vi "ArmEndEffectorPosition.vi"(2 "Wrist Angle (deg)":dbl, 3 "Elbow Angle (deg)":dbl, 4 "Shoulder Angle (deg)":dbl) -> (0 "Rotation Vector (deg)":cluster{"roll":dbl, "pitch":dbl, "yaw":dbl}, 1 "Translation Vector (in)":dbl[](array[numeric]))   [LabVIEW 2020]
doc: "Calculates the goal end effector position based on the goal arm joint angles."
uses:
  GlobalArm.vi
  <vilib>/robotics/Kinematics/Robot/Forward Kinematics (Point).vi
  <vilib>/robotics/Kinematics/NI_Kinematics.lvlib
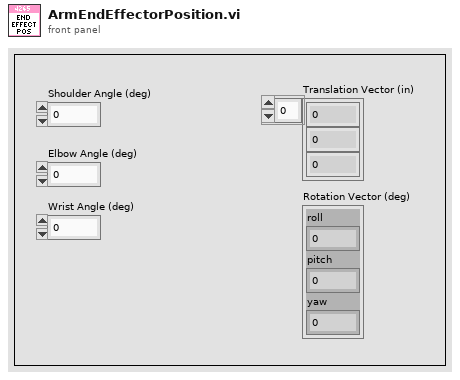
[diagram p1: front panel]
types:
  T1 = typedef "NI_Matrix.lvlib/RealMatrix.ctl" = dbl[][]
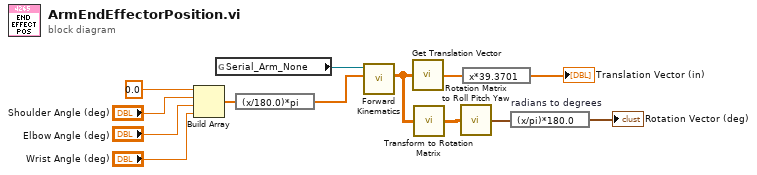
[diagram p0: block diagram]
diagram:
  n1 = Build Array(0.0 ("element"), "Shoulder Angle (deg)", "Elbow Angle (deg)", "Wrist Angle (deg)") -> (w12:dbl[])
  n2 = global read "GlobalArm.vi" "Serial_Arm_None"() -> (w7:refnum<class "NI_Robotics_Serial Robot Arm.lvclass">)
  n3 = expression code="(x/180.0)*pi" ("degrees to radians")(w12) -> (w13:dbl[])
  n4 = call-poly <vilib>:"Forward Kinematics.vi"("joint positions"=w13, "serial arm in"=w7) -> ("end effector transform"=w4:T1)  [unwired: 7 in, 2 out]
  n5 = call <vilib>:"Get Translation Vector.vi"("transform"=w4) -> ("translation vector"=w6:dbl[])
  n6 = call <vilib>:"Transform to Rotation Matrix.vi"("transform"=w4) -> ("rotation matrix"=w3:T1)
  n7 = call <vilib>:"Rotation Matrix to Roll Pitch Yaw.vi"("rotation matrix"=w3) -> ("angles"=w2:cluster{"roll":dbl, "pitch":dbl, "yaw":dbl})
  n8 = expression code="x*39.3701" ("degrees to radians")(w6) -> (→"Translation Vector (in)":dbl[])
  n9 = expression code="(x/pi)*180.0" "radians to degrees"(w2) -> (→"Rotation Vector (deg)":cluster{"roll":dbl, "pitch":dbl, "yaw":dbl})
